vi "cps_serial_write.vi"(0 "Dato da leggere":u16(ring) items=["Nessuno", "Tensione set", "Tensione out", "Corrente out", "Fase set", "Freq set", "Allarmi", "Modo", "Revisione e codice macchina", "Opzioni", "Fondo scala", "Banco forma onda"], 1 "Data (COM)":u16, 2 "Type (COM)":u16(ring) items=["REMOTO", "OUT", "RANGE", "SENSE", "MONO", "SINC", "DC", "INRUSH", "WAVEFORM"], 4 "Range L":dbl, 5 "Range H":dbl, 6 "rampa tensione frequenza":T2 {"tiporampa" items=["Tensione"=0, "Frequenza"=1, "Fase"=3]}, 7 "COMANDO":T3, 8 "rampa tensione frequenza all":T1, 9 "CODE":u8(ring) items=["NONE", "INIT", "ACQ", "SETMD", "RAMPAVF", "RAMPAPAR", "COMANDO"]) -> (3 "Pacchetto":string)   [LabVIEW 2019]
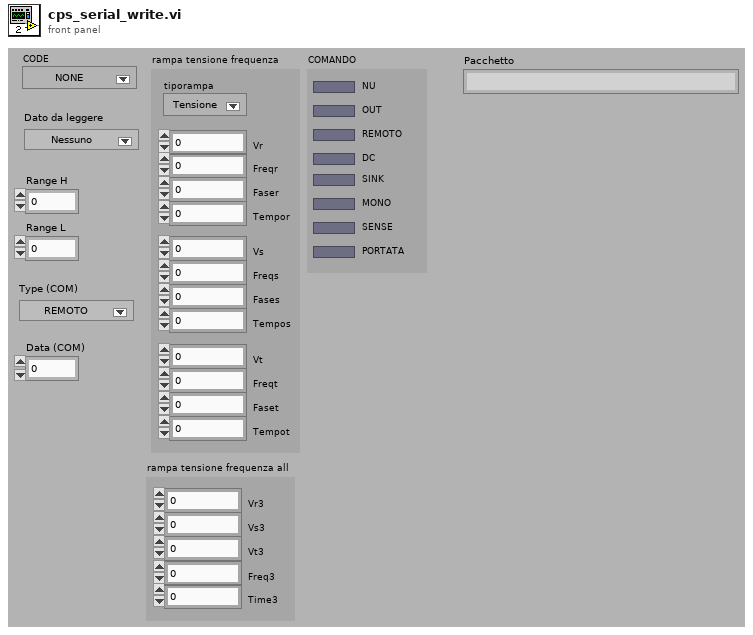
[diagram p1: front panel]
types:
  T1 = cluster{"Vr3":dbl, "Vs3":dbl, "Vt3":dbl, "Freq3":dbl, "Time3":dbl}
  T2 = cluster{"Vr":dbl, "Tempor":dbl, "Freqr":dbl, "Faser":dbl, "Vs":dbl, "Freqs":dbl, "Fases":dbl, "Tempos":dbl, "Vt":dbl, "Freqt":dbl, "Faset":dbl, "Tempot":dbl, "tiporampa":u8}
  T3 = cluster{"NU":bool, "OUT":bool, "REMOTO":bool, "DC":bool, "SINK":bool, "MONO":bool, "SENSE":bool, "PORTATA":bool}
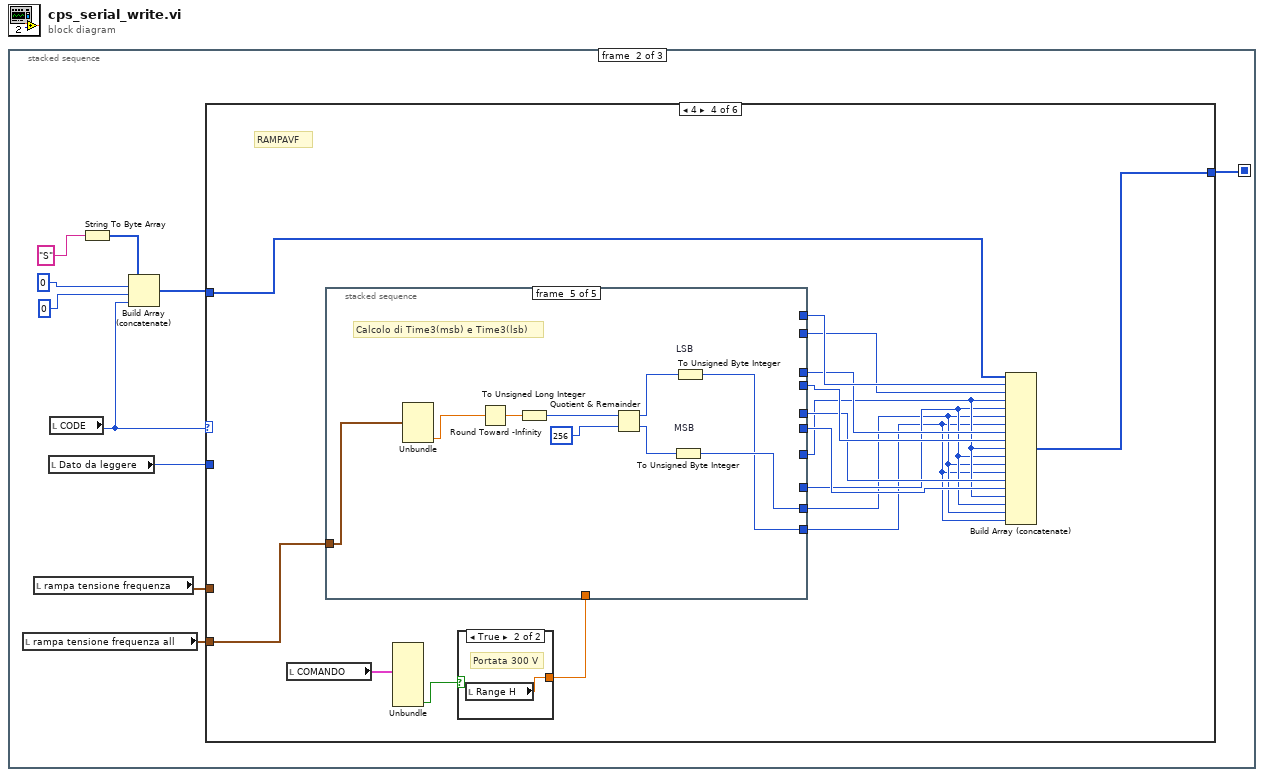
[diagram p0: block diagram]
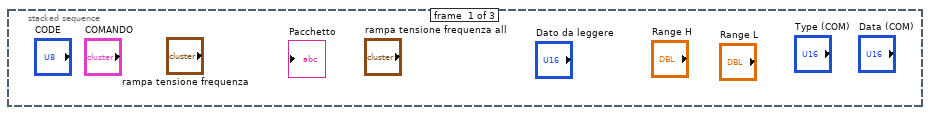
[diagram p2: hidden frame]
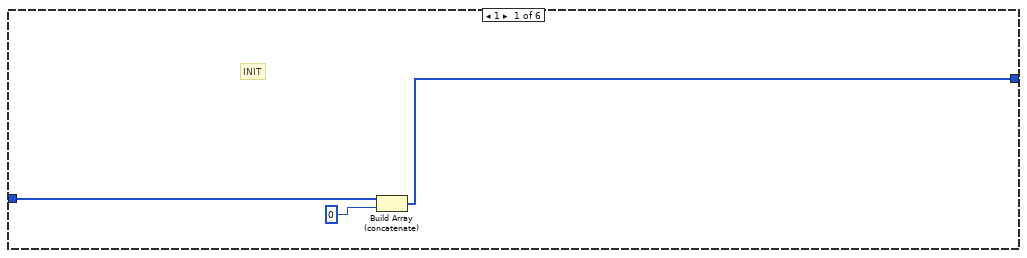
[diagram p3: hidden frame]
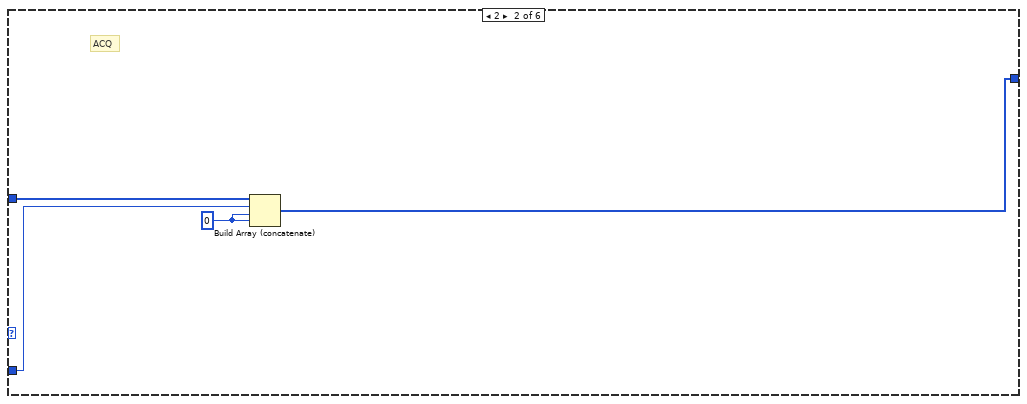
[diagram p4: hidden frame]
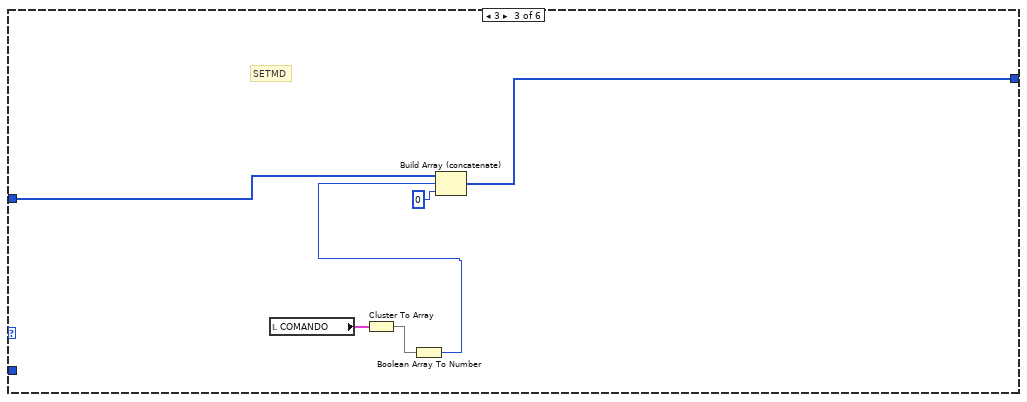
[diagram p5: hidden frame]
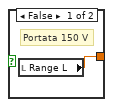
[diagram p6: hidden frame]
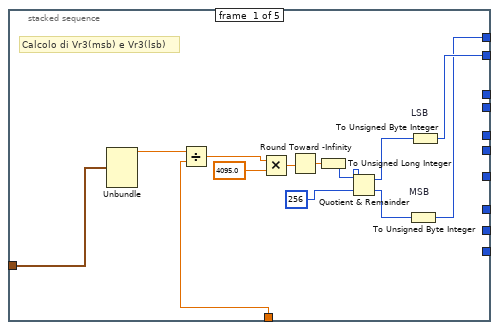
[diagram p7: hidden frame]
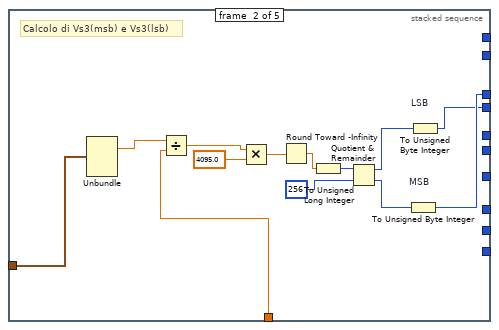
[diagram p8: hidden frame]
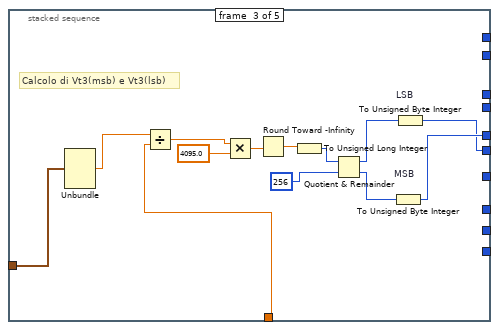
[diagram p9: hidden frame]
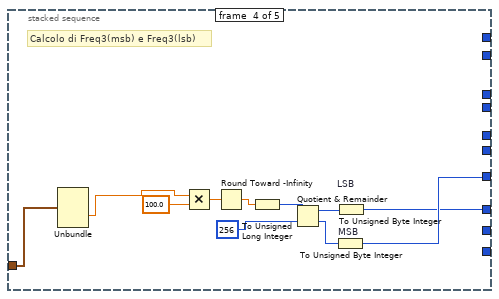
[diagram p10: hidden frame]
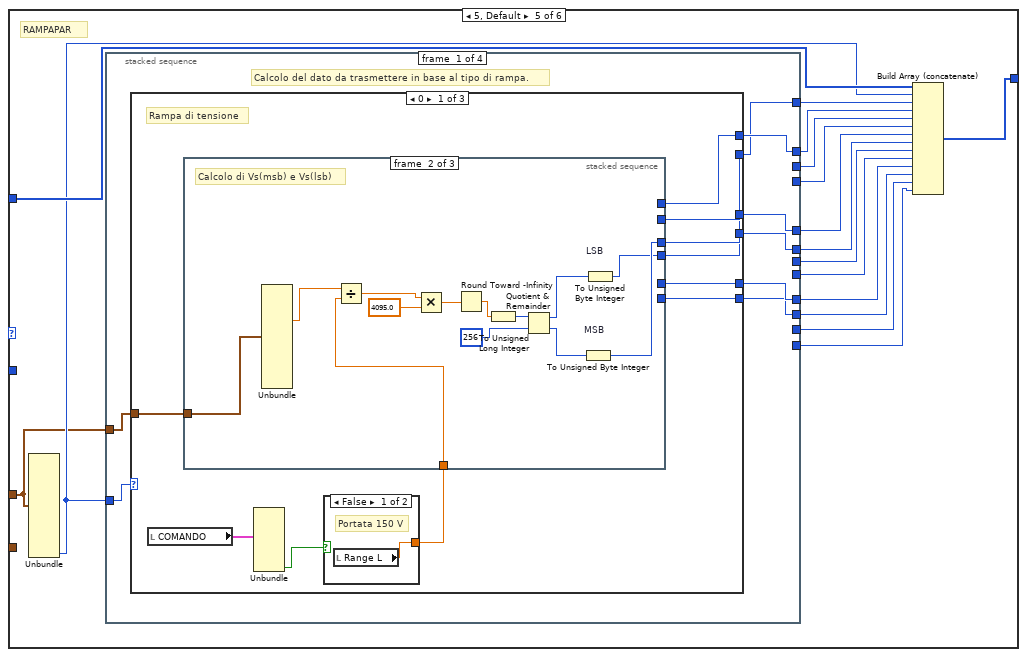
[diagram p11: hidden frame]
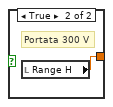
[diagram p12: hidden frame]
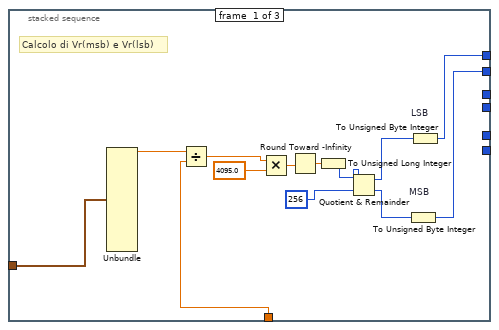
[diagram p13: hidden frame]
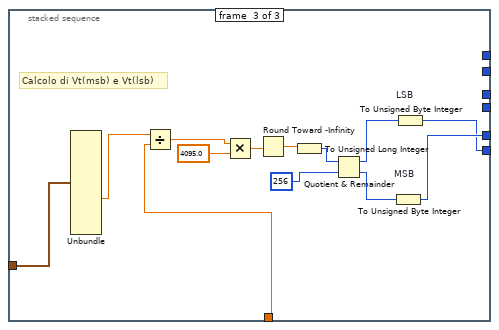
[diagram p14: hidden frame]
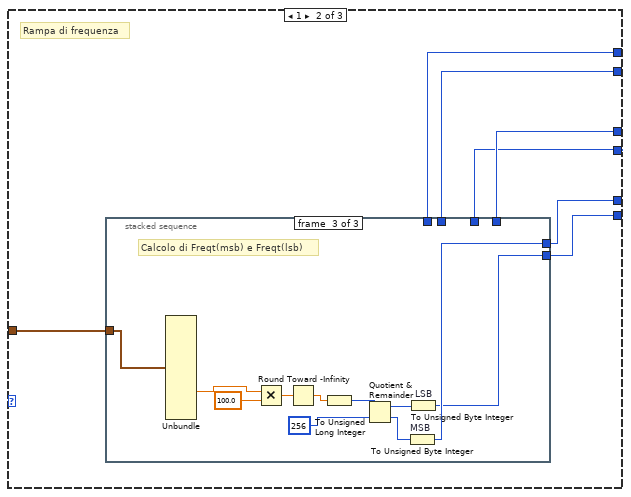
[diagram p15: hidden frame]
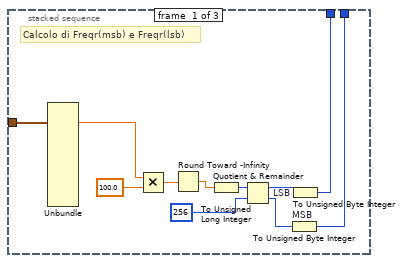
[diagram p16: hidden frame]
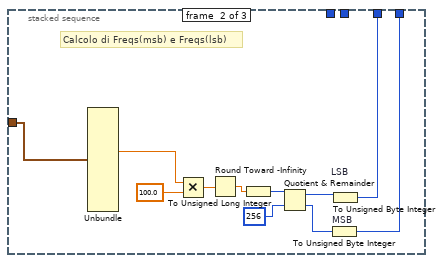
[diagram p17: hidden frame]
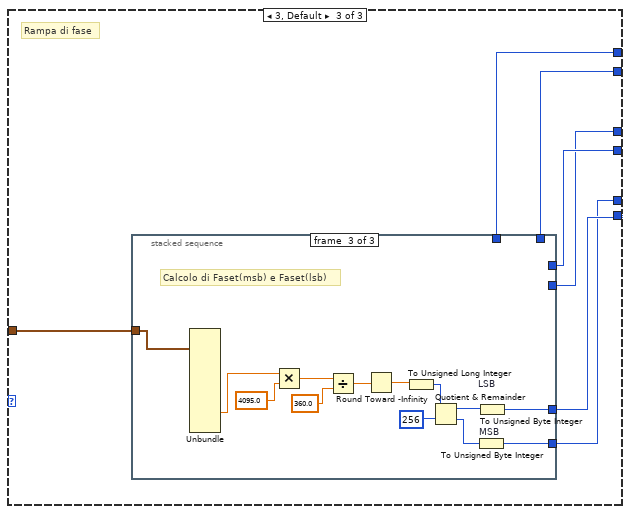
[diagram p18: hidden frame]
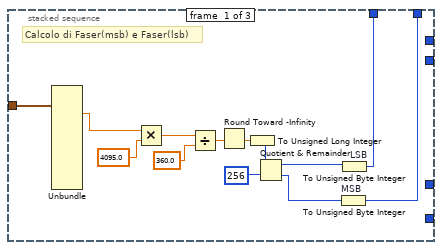
[diagram p19: hidden frame]
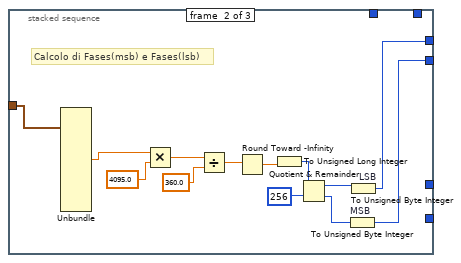
[diagram p20: hidden frame]
diagram:
  n1 = stacked-sequence {
    seq-local: [_ w5 _] -> [_ _ w294]
    frame #0 {
    }
    frame #1 {
      n2 = local read "rampa tensione frequenza all"() -> (w2:T1)
      n3 = local read "rampa tensione frequenza"() -> (w3:T2)
      n4 = local read "Dato da leggere"() -> (w1:u16)
      n5 = local read "CODE"() -> (w4:u8)
      n6 = String To Byte Array(string="S") -> (unsigned byte array=w10:u8[])
      n7 = Build Array (concatenate) "Build Array"(w10, u8 0 ("element"), u8 0 ("element"), w4) -> (w6:u8[])
      n8 = case shown="4" w4 {
        tunnel: [w12 w14 w18 w25 w116 w289] -> w5
        tunnel: w6 -> [w13 w17 w21 w24 w115 w292]
        tunnel: w3 -> [_ _ _ _ w107 _]
        tunnel: w2 -> [_ _ _ w39 _ _]
        tunnel: w1 -> [_ w16 _ _ _ _]
        frame 1 {
          # "INIT"
          n9 = Build Array (concatenate) "Build Array"(w13, u8 0 ("element")) -> (w12:u8[])
        }
        frame 2 {
          w15 = u16 0 ("element")
          # "ACQ"
          n10 = Build Array (concatenate) "Build Array"(w17, w16, w15, w15) -> (w14:u16[])
        }
        frame 3 {
          # "SETMD"
          n11 = local read "COMANDO"() -> (w23:T3)
          n12 = Cluster To Array(cluster=w23) -> (array=w22:bool[])
          n13 = Boolean Array To Number(Boolean array=w22) -> (number=w20:u32)
          n14 = Build Array (concatenate) "Build Array"(w21, w20, u8 0 ("element")) -> (w18:u32[])
        }
        frame 4 {
          # "RAMPAVF"
          n15 = local read "COMANDO"() -> (w38:T3)
          n16 = Unbundle "Unbundle"(w38) -> ("PORTATA"=w37:bool)  [unwired: 7 out]
          n17 = case shown="True" w37 {
            tunnel: [w40 w41] -> w36
            frame False {
              # "Portata 150 V"
              n18 = local read "Range L"() -> (w40:dbl)
            }
            frame True {
              # "Portata 300 V"
              n19 = local read "Range H"() -> (w41:dbl)
            }
          }
          n20 = stacked-sequence {
            tunnel: [w51 _ _ _ _] -> w34
            tunnel: [w50 _ _ _ _] -> w35
            tunnel: w39 -> [w46 w61 w69 w84 w95]
            tunnel: [_ w60 _ _ _] -> w33
            tunnel: [_ w59 _ _ _] -> w32
            tunnel: w36 -> [w44 w58 w74 _ _]
            tunnel: [_ _ w73 _ _] -> w31
            tunnel: [_ _ w72 _ _] -> w30
            tunnel: [_ _ _ w82 _] -> w29
            tunnel: [_ _ _ w81 _] -> w28
            tunnel: [_ _ _ _ w93] -> w27
            tunnel: [_ _ _ _ w92] -> w26
            frame #0 {
              # "Calcolo di Vr3(msb) e Vr3(lsb)"
              n21 = Unbundle "Unbundle"(w46) -> ("Vr3"=w53:dbl)  [unwired: 4 out]
              n22 = Divide(x=w53, y=w44) -> (x/y=w52:dbl)
              n23 = Multiply(x=w52, y=4095.0) -> (x*y=w43:dbl)
              n24 = Round Toward -Infinity(1:w43) -> (0:w42:dbl)
              n25 = To Unsigned Long Integer(number=w42) -> (unsigned 32bit integer=w48:u32)
              n26 = Quotient & Remainder(x=w48, y=u32 256) -> (x-y*floor(x/y)=w47:u32, floor(x/y)=w45:u32)
              n27 = To Unsigned Byte Integer "MSB"(number=w45) -> (unsigned 8bit integer=w50:u8)
              n28 = To Unsigned Byte Integer "LSB"(number=w47) -> (unsigned 8bit integer=w51:u8)
            }
            frame #1 {
              # "Calcolo di Vs3(msb) e Vs3(lsb)"
              n29 = Unbundle "Unbundle"(w61) -> ("Vs3"=w55:dbl)  [unwired: 4 out]
              n30 = Divide(x=w55, y=w58) -> (x/y=w63:dbl)
              n31 = Multiply(x=w63, y=4095.0) -> (x*y=w57:dbl)
              n32 = Round Toward -Infinity(1:w57) -> (0:w56:dbl)
              n33 = To Unsigned Long Integer(number=w56) -> (unsigned 32bit integer=w65:u32)
              n34 = Quotient & Remainder(x=w65, y=u32 256) -> (x-y*floor(x/y)=w66:u32, floor(x/y)=w67:u32)
              n35 = To Unsigned Byte Integer "MSB"(number=w67) -> (unsigned 8bit integer=w60:u8)
              n36 = To Unsigned Byte Integer "LSB"(number=w66) -> (unsigned 8bit integer=w59:u8)
            }
            frame #2 {
              # "Calcolo di Vt3(msb) e Vt3(lsb)"
              n37 = Unbundle "Unbundle"(w69) -> ("Vt3"=w68:dbl)  [unwired: 4 out]
              n38 = Divide(x=w68, y=w74) -> (x/y=w79:dbl)
              n39 = Multiply(x=w79, y=4095.0) -> (x*y=w71:dbl)
              n40 = Round Toward -Infinity(1:w71) -> (0:w70:dbl)
              n41 = To Unsigned Long Integer(number=w70) -> (unsigned 32bit integer=w77:u32)
              n42 = Quotient & Remainder(x=w77, y=u32 256) -> (x-y*floor(x/y)=w76:u32, floor(x/y)=w75:u32)
              n43 = To Unsigned Byte Integer "MSB"(number=w75) -> (unsigned 8bit integer=w73:u8)
              n44 = To Unsigned Byte Integer "LSB"(number=w76) -> (unsigned 8bit integer=w72:u8)
            }
            frame #3 {
              # "Calcolo di Freq3(msb) e Freq3(lsb)"
              n45 = Unbundle "Unbundle"(w84) -> ("Freq3"=w83:dbl)  [unwired: 4 out]
              n46 = Multiply(x=w83, y=100.0) -> (x*y=w90:dbl)
              n47 = Round Toward -Infinity(1:w90) -> (0:w91:dbl)
              n48 = To Unsigned Long Integer(number=w91) -> (unsigned 32bit integer=w86:u32)
              n49 = Quotient & Remainder(x=w86, y=u32 256) -> (x-y*floor(x/y)=w87:u32, floor(x/y)=w85:u32)
              n50 = To Unsigned Byte Integer "MSB"(number=w85) -> (unsigned 8bit integer=w82:u8)
              n51 = To Unsigned Byte Integer "LSB"(number=w87) -> (unsigned 8bit integer=w81:u8)
            }
            frame #4 {
              # "Calcolo di Time3(msb) e Time3(lsb)"
              n52 = Unbundle "Unbundle"(w95) -> ("Time3"=w94:dbl)  [unwired: 4 out]
              n53 = Round Toward -Infinity(1:w94) -> (0:w96:dbl)
              n54 = To Unsigned Long Integer(number=w96) -> (unsigned 32bit integer=w99:u32)
              n55 = Quotient & Remainder(x=w99, y=u32 256) -> (x-y*floor(x/y)=w98:u32, floor(x/y)=w97:u32)
              n56 = To Unsigned Byte Integer "MSB"(number=w97) -> (unsigned 8bit integer=w93:u8)
              n57 = To Unsigned Byte Integer "LSB"(number=w98) -> (unsigned 8bit integer=w92:u8)
            }
          }
          n58 = Build Array (concatenate) "Build Array"(w24, w35, w34, w29, w28, w27, w26, w33, w32, w29, w28, w27, w26, w31, w30, w29, w28, w27, w26) -> (w25:u8[])
        }
        frame 5, Default {
          # "RAMPAPAR"
          n59 = Unbundle "Unbundle"(w107) -> ("tiporampa"=w114:u8)  [unwired: 12 out]
          n60 = stacked-sequence {
            tunnel: w114 -> [w124 _ _ _]
            tunnel: [w123 _ _ _] -> w113
            tunnel: [w122 _ _ _] -> w112
            tunnel: [w121 _ _ _] -> w111
            tunnel: [w120 _ _ _] -> w110
            tunnel: [w119 _ _ _] -> w109
            tunnel: [w118 _ _ _] -> w108
            tunnel: w107 -> [w117 w266 w275 w284]
            tunnel: [_ w265 _ _] -> w106
            tunnel: [_ w264 _ _] -> w105
            tunnel: [_ _ w274 _] -> w104
            tunnel: [_ _ w273 _] -> w103
            tunnel: [_ _ _ w283] -> w102
            tunnel: [_ _ _ w282] -> w101
            frame #0 {
              # "Calcolo del dato da trasmettere in base al tipo di rampa."
              n61 = case shown="0" w124 {
                tunnel: [w134 w180 w221] -> w123
                tunnel: [w133 w181 w220] -> w122
                tunnel: w117 -> [w132 w182 w222]
                tunnel: [w131 w179 w218] -> w121
                tunnel: [w130 w178 w219] -> w120
                tunnel: [w126 w177 w216] -> w119
                tunnel: [w125 w176 w217] -> w118
                frame 0 {
                  # "Rampa di tensione"
                  n62 = local read "COMANDO"() -> (w128:T3)
                  n63 = Unbundle "Unbundle"(w128) -> ("PORTATA"=w129:bool)  [unwired: 7 out]
                  n64 = case shown="False" w129 {
                    tunnel: [w135 w136] -> w127
                    frame False {
                      # "Portata 150 V"
                      n65 = local read "Range L"() -> (w135:dbl)
                    }
                    frame True {
                      # "Portata 300 V"
                      n66 = local read "Range H"() -> (w136:dbl)
                    }
                  }
                  n67 = stacked-sequence {
                    tunnel: [w146 _ _] -> w134
                    tunnel: [w145 _ _] -> w133
                    tunnel: w132 -> [w141 w156 w169]
                    tunnel: [_ w155 _] -> w131
                    tunnel: [_ w154 _] -> w130
                    tunnel: w127 -> [w139 w152 w167]
                    tunnel: [_ _ w166] -> w126
                    tunnel: [_ _ w165] -> w125
                    frame #0 {
                      # "Calcolo di Vr(msb) e Vr(lsb)"
                      n68 = Unbundle "Unbundle"(w141) -> ("Vr"=w148:dbl)  [unwired: 12 out]
                      n69 = Divide(x=w148, y=w139) -> (x/y=w147:dbl)
                      n70 = Multiply(x=w147, y=4095.0) -> (x*y=w138:dbl)
                      n71 = Round Toward -Infinity(1:w138) -> (0:w137:dbl)
                      n72 = To Unsigned Long Integer(number=w137) -> (unsigned 32bit integer=w143:u32)
                      n73 = Quotient & Remainder(x=w143, y=u32 256) -> (x-y*floor(x/y)=w142:u32, floor(x/y)=w140:u32)
                      n74 = To Unsigned Byte Integer "MSB"(number=w140) -> (unsigned 8bit integer=w145:u8)
                      n75 = To Unsigned Byte Integer "LSB"(number=w142) -> (unsigned 8bit integer=w146:u8)
                    }
                    frame #1 {
                      # "Calcolo di Vs(msb) e Vs(lsb)"
                      n76 = Unbundle "Unbundle"(w156) -> ("Vs"=w153:dbl)  [unwired: 12 out]
                      n77 = Divide(x=w153, y=w152) -> (x/y=w158:dbl)
                      n78 = Multiply(x=w158, y=4095.0) -> (x*y=w151:dbl)
                      n79 = Round Toward -Infinity(1:w151) -> (0:w150:dbl)
                      n80 = To Unsigned Long Integer(number=w150) -> (unsigned 32bit integer=w160:u32)
                      n81 = Quotient & Remainder(x=w160, y=u32 256) -> (x-y*floor(x/y)=w161:u32, floor(x/y)=w162:u32)
                      n82 = To Unsigned Byte Integer "MSB"(number=w162) -> (unsigned 8bit integer=w155:u8)
                      n83 = To Unsigned Byte Integer "LSB"(number=w161) -> (unsigned 8bit integer=w154:u8)
                    }
                    frame #2 {
                      # "Calcolo di Vt(msb) e Vt(lsb)"
                      n84 = Unbundle "Unbundle"(w169) -> ("Vt"=w168:dbl)  [unwired: 12 out]
                      n85 = Divide(x=w168, y=w167) -> (x/y=w174:dbl)
                      n86 = Multiply(x=w174, y=4095.0) -> (x*y=w164:dbl)
                      n87 = Round Toward -Infinity(1:w164) -> (0:w163:dbl)
                      n88 = To Unsigned Long Integer(number=w163) -> (unsigned 32bit integer=w172:u32)
                      n89 = Quotient & Remainder(x=w172, y=u32 256) -> (x-y*floor(x/y)=w171:u32, floor(x/y)=w170:u32)
                      n90 = To Unsigned Byte Integer "MSB"(number=w170) -> (unsigned 8bit integer=w166:u8)
                      n91 = To Unsigned Byte Integer "LSB"(number=w171) -> (unsigned 8bit integer=w165:u8)
                    }
                  }
                }
                frame 1 {
                  # "Rampa di frequenza"
                  n92 = stacked-sequence {
                    tunnel: w182 -> [w193 w199 w210]
                    tunnel: [w189 _ _] -> w181
                    tunnel: [w188 _ _] -> w180
                    tunnel: [_ w197 _] -> w179
                    tunnel: [_ w196 _] -> w178
                    tunnel: [_ _ w208] -> w177
                    tunnel: [_ _ w207] -> w176
                    frame #0 {
                      # "Calcolo di Freqr(msb) e Freqr(lsb)"
                      n93 = Unbundle "Unbundle"(w193) -> ("Freqr"=w186:dbl)  [unwired: 12 out]
                      n94 = Multiply(x=w186, y=100.0) -> (x*y=w183:dbl)
                      n95 = Round Toward -Infinity(1:w183) -> (0:w184:dbl)
                      n96 = To Unsigned Long Integer(number=w184) -> (unsigned 32bit integer=w187:u32)
                      n97 = Quotient & Remainder(x=w187, y=u32 256) -> (x-y*floor(x/y)=w190:u32, floor(x/y)=w185:u32)
                      n98 = To Unsigned Byte Integer "MSB"(number=w185) -> (unsigned 8bit integer=w189:u8)
                      n99 = To Unsigned Byte Integer "LSB"(number=w190) -> (unsigned 8bit integer=w188:u8)
                    }
                    frame #1 {
                      # "Calcolo di Freqs(msb) e Freqs(lsb)"
                      n100 = Unbundle "Unbundle"(w199) -> ("Freqs"=w198:dbl)  [unwired: 12 out]
                      n101 = Multiply(x=w198, y=100.0) -> (x*y=w195:dbl)
                      n102 = Round Toward -Infinity(1:w195) -> (0:w194:dbl)
                      n103 = To Unsigned Long Integer(number=w194) -> (unsigned 32bit integer=w203:u32)
                      n104 = Quotient & Remainder(x=w203, y=u32 256) -> (x-y*floor(x/y)=w202:u32, floor(x/y)=w204:u32)
                      n105 = To Unsigned Byte Integer "MSB"(number=w204) -> (unsigned 8bit integer=w197:u8)
                      n106 = To Unsigned Byte Integer "LSB"(number=w202) -> (unsigned 8bit integer=w196:u8)
                    }
                    frame #2 {
                      # "Calcolo di Freqt(msb) e Freqt(lsb)"
                      n107 = Unbundle "Unbundle"(w210) -> ("Freqt"=w209:dbl)  [unwired: 12 out]
                      n108 = Multiply(x=w209, y=100.0) -> (x*y=w206:dbl)
                      n109 = Round Toward -Infinity(1:w206) -> (0:w205:dbl)
                      n110 = To Unsigned Long Integer(number=w205) -> (unsigned 32bit integer=w214:u32)
                      n111 = Quotient & Remainder(x=w214, y=u32 256) -> (x-y*floor(x/y)=w213:u32, floor(x/y)=w215:u32)
                      n112 = To Unsigned Byte Integer "MSB"(number=w215) -> (unsigned 8bit integer=w208:u8)
                      n113 = To Unsigned Byte Integer "LSB"(number=w213) -> (unsigned 8bit integer=w207:u8)
                    }
                  }
                }
                frame 3, Default {
                  # "Rampa di fase"
                  n114 = stacked-sequence {
                    tunnel: w222 -> [w235 w241 w254]
                    tunnel: [w228 _ _] -> w221
                    tunnel: [w227 _ _] -> w220
                    tunnel: [_ w239 _] -> w219
                    tunnel: [_ w238 _] -> w218
                    tunnel: [_ _ w252] -> w217
                    tunnel: [_ _ w251] -> w216
                    frame #0 {
                      # "Calcolo di Faser(msb) e Faser(lsb)"
                      n115 = Unbundle "Unbundle"(w235) -> ("Faser"=w226:dbl)  [unwired: 12 out]
                      n116 = Multiply(x=w226, y=4095.0) -> (x*y=w233:dbl)
                      n117 = Divide(x=w233, y=360.0) -> (x/y=w224:dbl)
                      n118 = Round Toward -Infinity(1:w224) -> (0:w223:dbl)
                      n119 = To Unsigned Long Integer(number=w223) -> (unsigned 32bit integer=w230:u32)
                      n120 = Quotient & Remainder(x=w230, y=u32 256) -> (x-y*floor(x/y)=w231:u32, floor(x/y)=w225:u32)
                      n121 = To Unsigned Byte Integer "MSB"(number=w225) -> (unsigned 8bit integer=w227:u8)
                      n122 = To Unsigned Byte Integer "LSB"(number=w231) -> (unsigned 8bit integer=w228:u8)
                    }
                    frame #1 {
                      # "Calcolo di Fases(msb) e Fases(lsb)"
                      n123 = Unbundle "Unbundle"(w241) -> ("Fases"=w240:dbl)  [unwired: 12 out]
                      n124 = Multiply(x=w240, y=4095.0) -> (x*y=w243:dbl)
                      n125 = Divide(x=w243, y=360.0) -> (x/y=w237:dbl)
                      n126 = Round Toward -Infinity(1:w237) -> (0:w236:dbl)
                      n127 = To Unsigned Long Integer(number=w236) -> (unsigned 32bit integer=w246:u32)
                      n128 = Quotient & Remainder(x=w246, y=u32 256) -> (x-y*floor(x/y)=w245:u32, floor(x/y)=w248:u32)
                      n129 = To Unsigned Byte Integer "MSB"(number=w248) -> (unsigned 8bit integer=w238:u8)
                      n130 = To Unsigned Byte Integer "LSB"(number=w245) -> (unsigned 8bit integer=w239:u8)
                    }
                    frame #2 {
                      # "Calcolo di Faset(msb) e Faset(lsb)"
                      n131 = Unbundle "Unbundle"(w254) -> ("Faset"=w253:dbl)  [unwired: 12 out]
                      n132 = Multiply(x=w253, y=4095.0) -> (x*y=w260:dbl)
                      n133 = Divide(x=w260, y=360.0) -> (x/y=w250:dbl)
                      n134 = Round Toward -Infinity(1:w250) -> (0:w249:dbl)
                      n135 = To Unsigned Long Integer(number=w249) -> (unsigned 32bit integer=w257:u32)
                      n136 = Quotient & Remainder(x=w257, y=u32 256) -> (x-y*floor(x/y)=w258:u32, floor(x/y)=w255:u32)
                      n137 = To Unsigned Byte Integer "MSB"(number=w255) -> (unsigned 8bit integer=w251:u8)
                      n138 = To Unsigned Byte Integer "LSB"(number=w258) -> (unsigned 8bit integer=w252:u8)
                    }
                  }
                }
              }
            }
            frame #1 {
              # "Calcolo di Tempor(msb) e Tempor(lsb)"
              n139 = Unbundle "Unbundle"(w266) -> ("Tempor"=w263:dbl)  [unwired: 12 out]
              n140 = Round Toward -Infinity(1:w263) -> (0:w262:dbl)
              n141 = To Unsigned Long Integer(number=w262) -> (unsigned 32bit integer=w269:u32)
              n142 = Quotient & Remainder(x=w269, y=u32 256) -> (x-y*floor(x/y)=w268:u32, floor(x/y)=w267:u32)
              n143 = To Unsigned Byte Integer "MSB"(number=w267) -> (unsigned 8bit integer=w265:u8)
              n144 = To Unsigned Byte Integer "LSB"(number=w268) -> (unsigned 8bit integer=w264:u8)
            }
            frame #2 {
              # "Calcolo di Tempos(msb) e Tempos(lsb)"
              n145 = Unbundle "Unbundle"(w275) -> ("Tempos"=w272:dbl)  [unwired: 12 out]
              n146 = Round Toward -Infinity(1:w272) -> (0:w271:dbl)
              n147 = To Unsigned Long Integer(number=w271) -> (unsigned 32bit integer=w278:u32)
              n148 = Quotient & Remainder(x=w278, y=u32 256) -> (x-y*floor(x/y)=w277:u32, floor(x/y)=w276:u32)
              n149 = To Unsigned Byte Integer "MSB"(number=w276) -> (unsigned 8bit integer=w274:u8)
              n150 = To Unsigned Byte Integer "LSB"(number=w277) -> (unsigned 8bit integer=w273:u8)
            }
            frame #3 {
              # "Calcolo di Tempot(msb) e Tempot(lsb)"
              n151 = Unbundle "Unbundle"(w284) -> ("Tempot"=w281:dbl)  [unwired: 12 out]
              n152 = Round Toward -Infinity(1:w281) -> (0:w280:dbl)
              n153 = To Unsigned Long Integer(number=w280) -> (unsigned 32bit integer=w287:u32)
              n154 = Quotient & Remainder(x=w287, y=u32 256) -> (x-y*floor(x/y)=w286:u32, floor(x/y)=w285:u32)
              n155 = To Unsigned Byte Integer "MSB"(number=w285) -> (unsigned 8bit integer=w283:u8)
              n156 = To Unsigned Byte Integer "LSB"(number=w286) -> (unsigned 8bit integer=w282:u8)
            }
          }
          n157 = Build Array (concatenate) "Build Array"(w115, w114, w112, w113, w106, w105, w111, w110, w104, w103, w109, w108, w102, w101) -> (w116:u8[])
        }
        frame 6 {
          # "COM"
          n158 = local read "Type (COM)"() -> (w291:u16)
          n159 = local read "Data (COM)"() -> (w290:u16)
          n160 = Build Array (concatenate)(w292, w291, w290) -> (w289:u16[])
        }
      }
    }
    frame #2 {
      w299 = 0 ("y")
      n161 = Array Size(array=w294) -> (size(s)=w301:i32)
      n162 = Add(x=w301, y=1) -> (x+y=w296:i32)
      n163 = Subtract(x=w301, y=4) -> (x-y=w297:i32)
      n164 = for {
        N: w297 -> [_]
        tunnel: w294 -> [w311]
        shift-right: [w308] -> w302
        shift-left: w299 -> [w309]
        i -> [w307]
        n165 = Add(x=4, y=w307) -> (x+y=w305:i32)
        n166 = Index Array "Index Array"(array=w311, index=w305) -> (element=w310:u32)
        n167 = Add(x=w310, y=w309) -> (x+y=w308:u32)
      }
      n168 = Build Array (concatenate) "Build Array"(w294, w302) -> (w303:u32[])
      n169 = for {
        N: w296 -> [_]
        shift-right: [w312] -> w304
        shift-left: w299 -> [w313]
        tunnel: w303 -> [w314]
        i -> [w316]
        n170 = Index Array "Index Array"(array=w314, index=w316) -> (element=w315:u32)
        n171 = Add(x=w315, y=w313) -> (x+y=w312:u32)
      }
      n172 = Build Array (concatenate) "Build Array"(w303, w304) -> (w300:u32[])
      n173 = Byte Array To String(unsigned byte array=w300) -> (string=w293:string)
      n174 = local write "Pacchetto"(w293) -> ()
    }
  }
